vi "Import Addon Configuration.vi"(8 "error in (no error)":errorcluster, 10 "configuration file path":path, 11 "FPGA Addon refnum in":T1=18446744073709551615 format="%.0x") -> (0 "error out":errorcluster, 3 "FPGA Addon refnum out":T1=18446744073709551615 format="%.0x")   [LabVIEW 2018, in "Scripting API.lvlib"]
uses:
  Scripting API.lvlib
  <vilib>/NI Veristand/Custom Device API/Custom Device Item Ref.ctl
  Addon/Addon Shared/Types/FG Action.ctl
  Addon/Addon Shared/Types/FPGA Settings.ctl
  Addon/Addon Shared/SubVIs/Constants.vi
  <vilib>/NI Veristand/Custom Device API/NI VeriStand - Get Item Property.vi
  <vilib>/NI Veristand/Custom Device API/Get Item Property (Path).vi
  <vilib>/NI Veristand/Custom Device API/Get Item Property (String).vi
  <vilib>/NI Veristand/Custom Device API/Get Item Property (Boolean).vi
  <vilib>/NI Veristand/Custom Device API/NI VeriStand - Set Item Property.vi
  <vilib>/NI Veristand/Custom Device API/Set Item Property (Path).vi
  <vilib>/NI Veristand/Custom Device API/Set Item Property (String).vi
  <vilib>/NI Veristand/Custom Device API/Set Item Property (Boolean).vi
  <vilib>/NI/NI VeriStand Custom Device Import and Export Tool/ImportExport.lvlib
  Addon/Addon Shared/FPGA Addon Shared.lvlib
  <vilib>/NI Veristand/Custom Device API/Custom Device API.lvlib
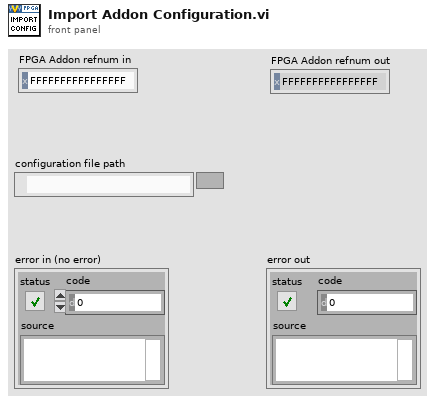
[diagram p1: front panel]
types:
  T1 = typedef "Custom Device API.lvlib/Custom Device Item Ref.ctl" = u64
  T2 = typedef "FPGA Addon Shared.lvlib/FPGA Settings.ctl" = cluster{"Bitfile path":path, "RIO Device Address":string, "Group":bool}
  T3 = typedef "FPGA Addon Shared.lvlib/FG Action.ctl" = enum8{"GET", "SET"}
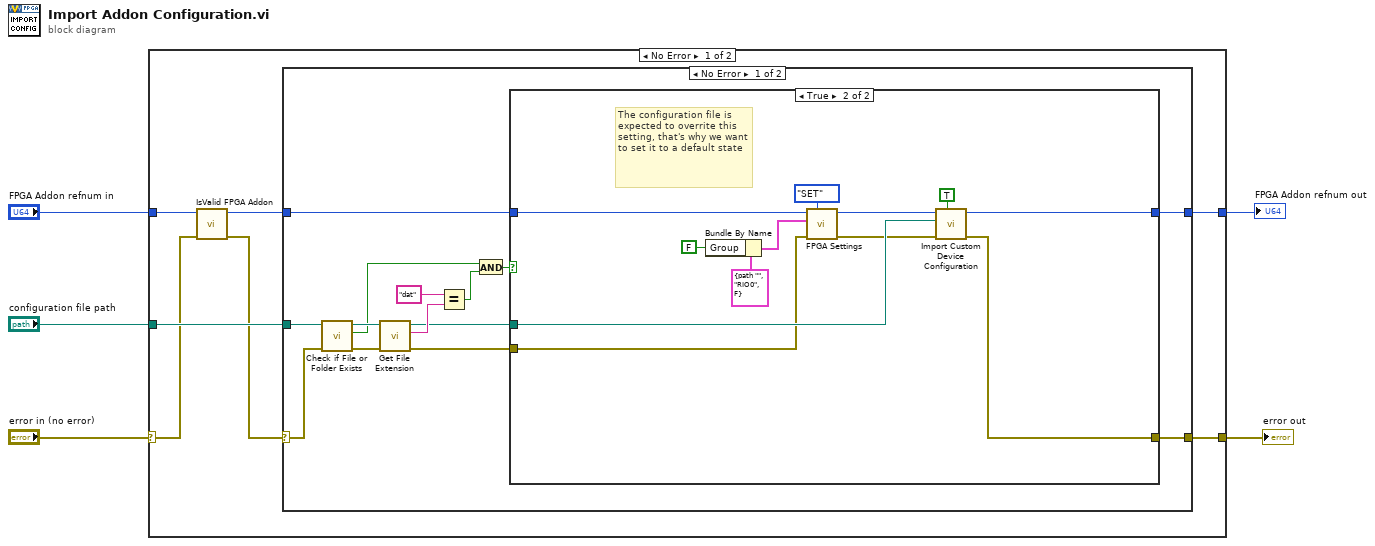
[diagram p0: block diagram]
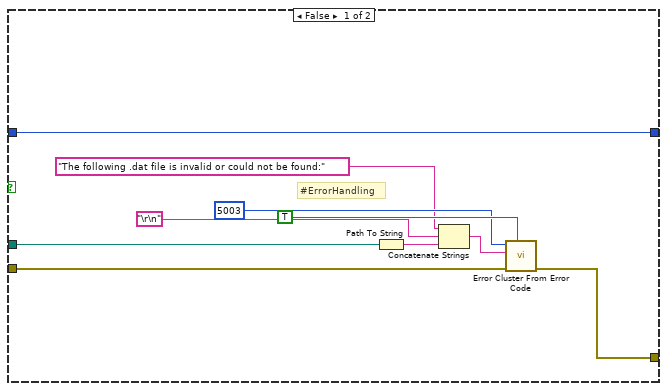
[diagram p2: hidden frame]
diagram:
  n1 = case shown="No Error" "error in (no error)" {
    selector: "error in (no error)" -> [w10 w51]
    tunnel: "FPGA Addon refnum in" -> [w12 w52]
    tunnel: "configuration file path" -> [w11 _]
    tunnel: [w8 w52] -> w2
    tunnel: [w7 w51] -> w1
    frame No Error {
      n2 = call "IsValid FPGA Addon.vi"("error in (no error)"=w10, "FPGA Addon refnum in"=w12) -> ("error out"=w6:errorcluster, "FPGA Addon refnum out"=w9:T1)  [unwired: 8 in]
      n3 = case shown="No Error" w6 {
        selector: w6 -> [w15 w50]
        tunnel: w11 -> [w21 _]
        tunnel: w9 -> [w20 w49]
        tunnel: [w18 w49] -> w8
        tunnel: [w17 w50] -> w7
        frame No Error {
          n4 = call <vilib>:"Check if File or Folder Exists.vi"("error in (no error)"=w15, "path"=w21) -> ("error out"=w26:errorcluster, "file or folder exists?"=w24:bool, "dup path"=w25:path)  [unwired: 7 in]
          n5 = call <vilib>:"Get File Extension.vi"("error in (no error)"=w26, "file"=w25) -> ("error out"=w19:errorcluster, "lowercase file extension"=w14:string, "dup file"=w13:path)  [unwired: 5 in, 2 out]
          n6 = Equal?(x="dat", y=w14) -> (x = y?=w22:bool)
          n7 = And(x=w24, y=w22) -> (x .and. y?=w16:bool)
          n8 = case shown="True" w16 {
            tunnel: w20 -> [w30 w41]
            tunnel: w19 -> [w29 w39]
            tunnel: [w30 w47] -> w18
            tunnel: [w28 w46] -> w17
            tunnel: w13 -> [w27 w45]
            frame False {
              # "#ErrorHandling"
              n9 = Path To String(path=w27) -> (string=w35:string)
              n10 = Concatenate Strings("The following .dat file is invalid or could not be found:" ("error message (\"\")"), "\r\n", w35) -> (w36:string)
              n11 = call <vilib>:"Error Cluster From Error Code.vi"("show call chain? (False)"=TRUE, "error in (no error)"=w29, "error message (\"\")"=w36, "error code (0)"=5003) -> ("error out"=w28:errorcluster)  [unwired: 5 in]
            }
            frame True {
              # "The configuration file is expected to overrite this setting, that's why we want to set it to a default state"
              n12 = Bundle By Name(cluster=T2 {"Bitfile path"=path "", "RIO Device Address"="RIO0", "Group"=FALSE} ("FPGA Settings"), "Group"=FALSE) -> (w44:T2)
              n13 = call "FPGA Settings.vi"("Action"=FG_Action."SET", "error in (no error)"=w39, "FPGA Settings"=w44, "Item Ref"=w41) -> ("error out"=w37:errorcluster, "Item Ref out"=w38:T1)  [unwired: 5 in, 1 out]
              n14 = call <vilib>:"Import Custom Device Configuration.vi"("Overwrite Existing?"=TRUE, "error in (no error)"=w37, "Path"=w45, "NodeID"=w38) -> ("error out"=w46:errorcluster, "NodeID out"=w47:u64)  [unwired: 5 in, 1 out]
            }
          }
        }
        frame Error {
        }
      }
    }
    frame Error {
    }
  }
  "error out" <- w1
  "FPGA Addon refnum out" <- w2
